vi "Find Topmost Match.vi"(10 "Name":string, 11 "Tree":variant) -> (1 "Found?":bool, 2 "Match":variant)   [LabVIEW 2019, in "Tree.lvclass"]
uses:
  Tree.lvclass
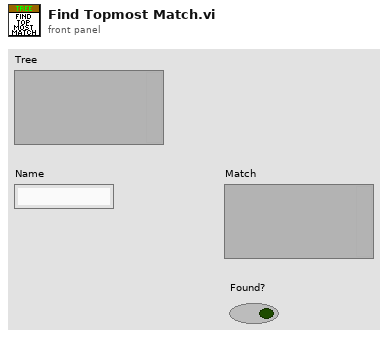
[diagram p1: front panel]
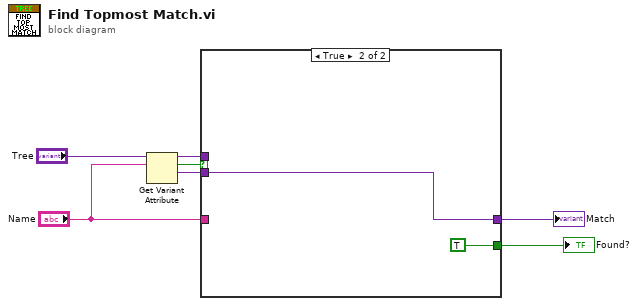
[diagram p0: block diagram]
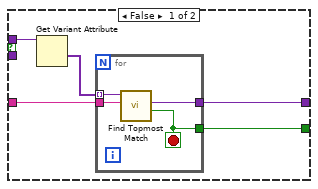
[diagram p2: hidden frame]
diagram:
  n1 = Get Variant Attribute(Variant="Tree", name="Name") -> (duplicate Variant=w7:variant, found=w6:bool, value=w3:variant)  [unwired: 2 in, 1 out]
  n2 = case shown="True" w6 {
    tunnel: w7 -> [w12 _]
    tunnel: "Name" -> [w10 _]
    tunnel: w3 -> [_ w18]
    tunnel: [w9 w18] -> w2
    tunnel: [w8 TRUE ("Found?")] -> w1
    frame False {
      n3 = Get Variant Attribute(Variant=w12) -> (values=w11:variant[])  [unwired: 3 in, 3 out]
      n4 = for {
        tunnel: w11 -> [w16] mode=indexing
        tunnel: w10 -> [w15]
        tunnel: [w14] -> w9
        tunnel: [w13] -> w8
        stop <- w13 stop-if-true
        n5 = call "Find Topmost Match.vi"("Name"=w15, "Tree"=w16) -> ("Found?"=w13:bool, "Match"=w14:variant)  [unwired: 8 in]
      }
    }
    frame True {
    }
  }
  "Found?" <- w1
  "Match" <- w2
